vi "YKWT500 Display Num Format.vi"(8 "error in (no error)":errorcluster, 10 "Display Format (0: Numeric)":u16(ring) items=["VAL4", "VAL8", "VAL16", "MATRIX", "ALL"], 11 "VISA resource name":refnum<visa-resource-name>="WT500") -> (0 "error out":errorcluster, 3 "VISA resource name out":refnum<visa-resource-name>)   [LabVIEW 2012]
doc: "This VI sends the Display Format Configuration command to the WT500."
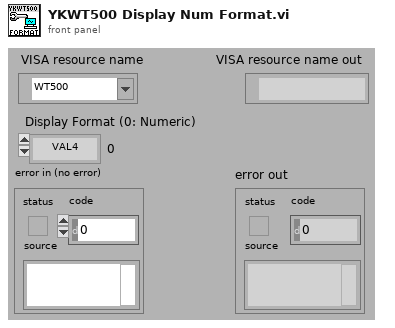
[diagram p1: front panel]
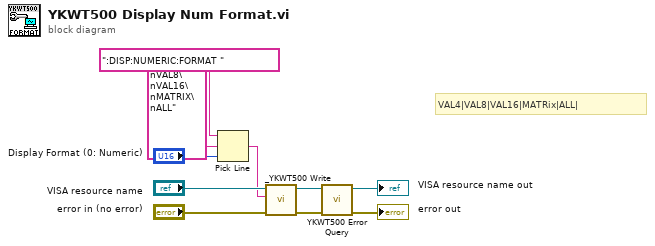
[diagram p0: block diagram]
diagram:
  # "VAL4|VAL8|VAL16|MATRix|ALL|"
  n1 = Pick Line(string ("")=":DISP:NUMERIC:FORMAT ", multi-line string="VAL4\nVAL8\nVAL16\nMATRIX\nALL", line index="Display Format (0: Numeric)") -> (output string=w5:string)
  n2 = call "_YKWT500 Write.vi"("error in (no error)"="error in (no error)", "Write Data"=w5, "VISA resource name"="VISA resource name") -> ("error out"=w3:errorcluster, "VISA resource name out"=w4:refnum<visa-resource-name>)  [unwired: 5 in, 2 out]
  n3 = call "YKWT500 Error Query.vi"("error in (no error)"=w3, "VISA resource name"=w4) -> ("error out"=→"error out":errorcluster, "VISA resource name out"=→"VISA resource name out":refnum<visa-resource-name>)  [unwired: 6 in, 2 out]
